vi "path name select.vi"(1 "NodePathArray":string[](array[string])) -> (0 "Label":string)   [LabVIEW 2011]
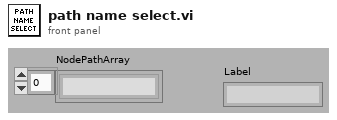
[diagram p1: front panel]
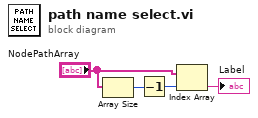
[diagram p0: block diagram]
diagram:
  n1 = Array Size(array="NodePathArray") -> (size(s)=w3:i32)
  n2 = Decrement(x=w3) -> (x-1=w2:i32)
  n3 = Index Array(array="NodePathArray", index=w2) -> (element=→"Label":string)
